vi "Get visa 1d DBL data.vi"(7 "VISA resource name":refnum<visa-resource-name>, 8 "error in (no error)":errorcluster, 9 "Name":string, 10 "Mag Lab Parameters in":refnum<class "Mag Lab Parameters.lvclass">, 11 "Oxford Power Supply in":refnum<class "Oxford Power Supply.lvclass">) -> (0 "error out":errorcluster, 1 "Channel data":dbl[](array[numeric]), 2 "Channel names":string[](array[string]), 3 "Oxford Power Supply out":refnum<class "Oxford Power Supply.lvclass">, 5 "VISA resource name out":refnum<visa-resource-name>)   [LabVIEW 2015, in "Oxford Power Supply.lvclass"]
uses:
  Oxford Power Supply.lvclass
  Mag Lab Properties/Mag Lab Parameters.lvclass
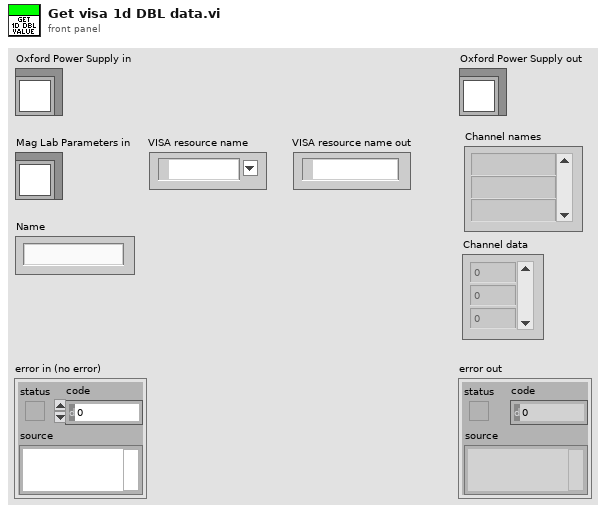
[diagram p1: front panel]
types:
  T1 = enum16{"open", "replace", "create", "open or create", "replace or create", "replace or create with confirmation"}
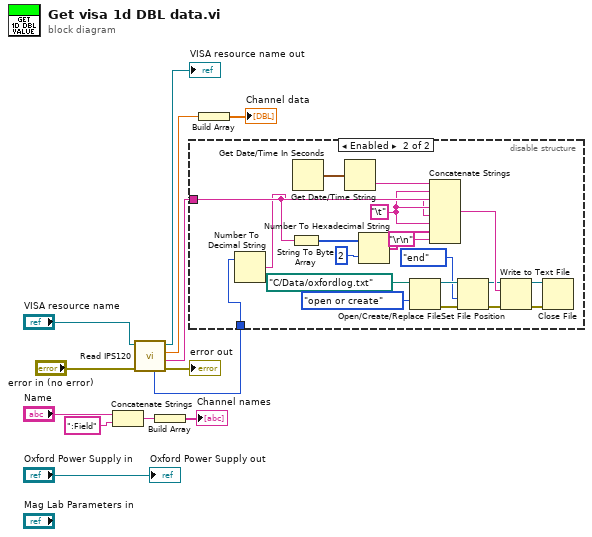
[diagram p0: block diagram]
diagram:
  n1 = Concatenate Strings("Name", ":Field" ("string")) -> (w6:string)
  n2 = call "Read IPS120.vi"("error in (no error)"="error in (no error)", "VISA resource name"="VISA resource name") -> ("error out"=→"error out":errorcluster, "read buffer"=w2:string, "Value"=w4:dbl, "VISA resource name out"=→"VISA resource name out":refnum<visa-resource-name>, "Repeats"=w1:i32)  [unwired: 5 in]
  n3 = Build Array(w6) -> (→"Channel names":string[])
  n4 = disable-structure shown="Enabled" {
    disable-tunnel: w2 -> [_ w22]
    disable-tunnel: w1 -> [_ w16]
    frame Disabled {
    }
    frame Enabled {
      w17 = "\t"
      n5 = Number To Decimal String(number=w16) -> (decimal integer string=w15:string)  [unwired: 1 in]
      n6 = String To Byte Array(string=w22) -> (unsigned byte array=w20:u8[])
      n7 = Get Date/Time In Seconds() -> (seconds since 1Jan1904=w24:timestamp)
      n8 = Get Date/Time String(seconds (now)=w24) -> (time string=w23:string)  [unwired: 2 in, 1 out]
      n9 = Number To Hexadecimal String(1:i16 2 ("width (-)"), 2:w20) -> (0:w19:string[])
      n10 = Open/Create/Replace File(file path (use dialog)=path "C:/Data/oxfordlog.txt", operation (0:open)=T1."open or create") -> (refnum out=w31:refnum<file>, error out=w30:errorcluster)  [unwired: 4 in, 1 out]
      n11 = Concatenate Strings(w23, w17, w22, w17, w15, w17, w19, "\r\n") -> (w33:string)
      n12 = Set File Position(refnum=w31, from (0:start)=enum16{"start", "end", "current"}."end", error in=w30) -> (refnum out=w27:refnum<file>, error out=w29:errorcluster)  [unwired: 1 in]
      n13 = Write to Text File(file (use dialog)=w27, text=w33, error in=w29) -> (refnum out=w25:refnum<file>, error out=w26:errorcluster)  [unwired: 1 in, 1 out]
      n14 = Close File(refnum=w25, error in=w26) -> ()  [unwired: 2 out]
    }
  }
  n15 = Build Array(w4) -> (→"Channel data":dbl[])
  "Oxford Power Supply out" <- "Oxford Power Supply in"
